vi "AnimateIntersection.vi"() -> ()   [LabVIEW 2022 SP3]
uses:
  <vilib>/Platform/NI_3dgraph.lvlib
panel:
  in  "delay":u32=10
  in  "Type Int":u16(ring) items=["Circle", "Plane"]
  in  "file name":string
  in  "save image":bool
  out "frame#":i32
  in  "Variables":T1={"sound spd (cm/s)"=150000, "time step (s)"=5e-07} {"time step (s)" format="%.2e"}
  in  "rotate P to -y":bool
  in  "Ring":i32(ring)=3 items=["Spherical cap", "Center Strip", "Half Sphere", "Wedge"]
  out "Output Cluster":T2 {"r5" format="%.2f"; "r4" format="%.4f"; "r3" format="%.4f"; "r2" format="%.4f"; "r1" format="%.4f"; "r0" format="%.2f"}
  in  "strip":cluster{"radius":dbl, "h":dbl, "a":dbl}={"radius"=4.0, "h"=0.5, "a"=3.0} {"radius" format="%.2f"; "a" format="%.2f"; "h" format="%.2f"}
  in  "P":cluster{"x":dbl, "y":dbl, "z":dbl}={"x"=0.2, "y"=-1.0, "z"=0.2} {"x" format="%.2f"; "z" format="%.2f"; "y" format="%.2f"}
  in  "ct sphere":cluster{"radius":dbl, "theta":dbl, "phi":dbl}={"radius"=10.0, "theta"=160.0, "phi"=100.0} {"radius" format="%.2f"; "phi" format="%.2f"; "theta" format="%.2f"}
  in  "3D Parametric Surface":refnum<k7>(container)
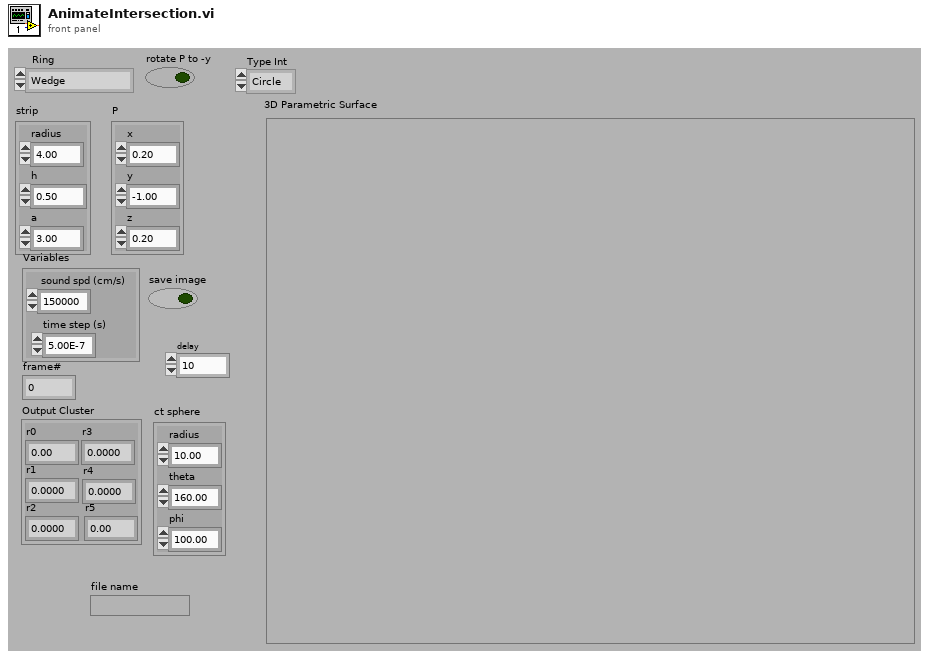
[diagram p1: front panel]
types:
  T1 = cluster{"sound spd (cm/s)":i32, "time step (s)":sgl}
  T2 = cluster{"r0":dbl, "r1":dbl, "r2":dbl, "r3":dbl, "r4":dbl, "r5":dbl}
  T3 = cluster{"r (cm)":dbl, "phih":dbl, "thetaw":dbl, "A":dbl, "B":dbl, "Dtemp":dbl}
  T4 = cluster{"alpha":bool, "beta":bool, "theta":bool, "phi":bool}
  T5 = typedef "LVRectTypeDef.ctl" = cluster{"left":i16, "top":i16, "right":i16, "bottom":i16}
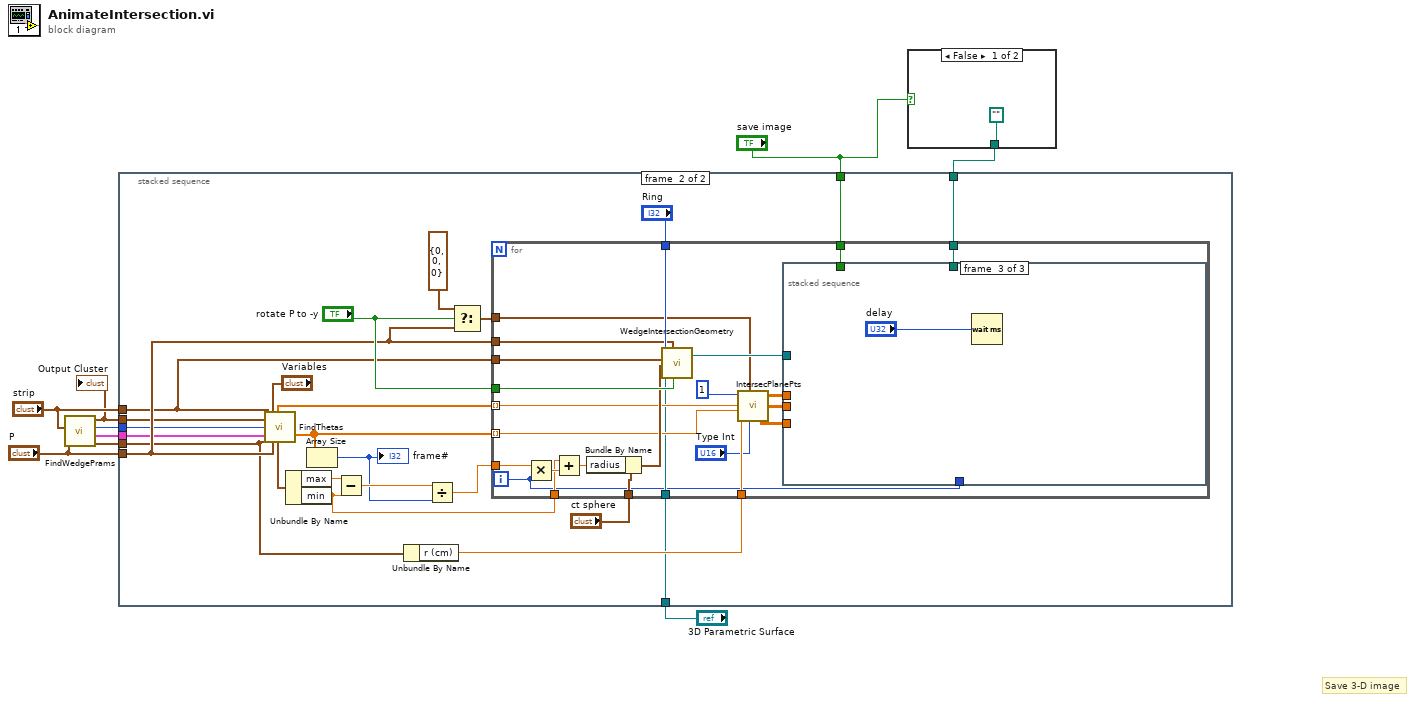
[diagram p0: block diagram]
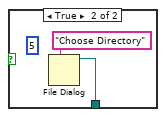
[diagram p2: hidden frame]
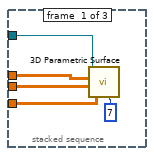
[diagram p4: hidden frame]
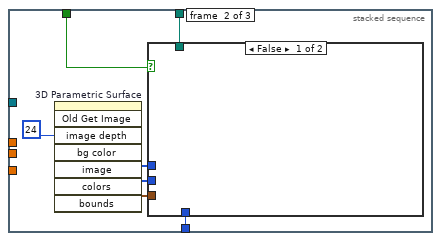
[diagram p5: hidden frame]
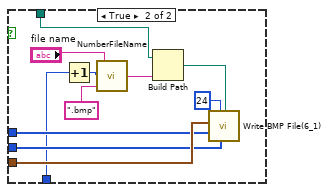
[diagram p6: hidden frame]
diagram:
  # "Save 3-D image"
  n1 = call "FindWedgePrams.vi"("P"="P", "strip"="strip") -> ("variables"=w4:T3, "Location Tests"=w6:T4, "Case Number"=w5:i32, "r values (cm)"=w3:T2)  [unwired: 2 in, 1 out]
  "Output Cluster" <- w3
  n2 = case shown="False" "save image" {
    tunnel: [path "" w11] -> w1
    frame False {
    }
    frame True {
      (unwired) 5
      n3 = File Dialog(7:"Choose Directory") -> (3:w11:path)  [unwired: 6 in, 3 out]
    }
  }
  n4 = stacked-sequence {
    tunnel: "P" -> [_ w22]
    tunnel: "strip" -> [_ w20]
    tunnel: "3D Parametric Surface" -> [_ w19]
    tunnel: w3 -> [_ w18]
    tunnel: w6 -> [_ w17]
    tunnel: w5 -> [_ w16]
    tunnel: w4 -> [_ w15]
    tunnel: "save image" -> [_ w14]
    tunnel: w1 -> [_ w13]
    frame #0 {
    }
    frame #1 {
      n5 = call "FindThetas.vi"("strip"=w20, "r values (cm)"=w18, "Case Number"=w16, "Location Tests"=w17, "P constants"=w15, "Variables"="Variables", "P (cm)"=w22) -> ("d"=w31:dbl[], "min/max r"=w36:cluster{"max":dbl, "min":dbl}, "sigma"=w30:dbl[])  [unwired: 2 in, 8 out]
      n6 = Unbundle By Name(w36) -> ("max"=w35:dbl, "min"=w32:dbl)
      n7 = Array Size(array=w30) -> (size(s)=w27:i32)
      "frame#" <- w27
      n8 = Subtract(x=w35, y=w32) -> (x-y=w34:dbl)
      n9 = Unbundle By Name(w15) -> ("r (cm)"=w21:dbl)
      n10 = Divide(x=w34, y=w27) -> (x/y=w33:dbl)
      n11 = Select(t=cluster{"radius":i32, "theta":i32, "phi":i32} {"radius"=0, "theta"=0, "phi"=0} ("ct sphere"), s="rotate P to -y", f=w22) -> (s? t:f=w29:cluster{"x":dbl, "y":dbl, "z":dbl})
      n12 = for {
        tunnel: w33 -> [w60]
        tunnel: w32 -> [w58]
        tunnel: w31 -> [w47] mode=indexing
        tunnel: w21 -> [w46]
        tunnel: w30 -> [w48] mode=indexing
        tunnel: w29 -> [w49]
        tunnel: "Ring" -> [w57]
        tunnel: w22 -> [w56]
        tunnel: w20 -> [w55]
        tunnel: "rotate P to -y" -> [w54]
        tunnel: "ct sphere" -> [w53]
        tunnel: w19 -> [w41]
        tunnel: w14 -> [w39]
        tunnel: w13 -> [w38]
        i -> [w40]
        n13 = Multiply(x=w60, y=w40) -> (x*y=w59:dbl)
        n14 = Add(x=w58, y=w59) -> (x+y=w52:dbl)
        n15 = Bundle By Name(cluster=w53, "radius"=w52) -> (w51:cluster{"radius":dbl, "theta":dbl, "phi":dbl})
        n16 = call "WedgeIntersectionGeometry.vi"("rotate P to -y"=w54, "P"=w56, "3D Parametric Surface"=w41, "ct sphere"=w51, "strip"=w55, "Ring"=w57) -> ("3D graph out"=w50:refnum<k7>)  [unwired: 1 in]
        n17 = call "IntersecPlanePts.vi"("circles"=1, "P"=w49, "d"=w47, "Sigma"=w48, "Ring"="Type Int", "r"=w46) -> ("x matrix"=w45:dbl[][], "y matrix"=w44:dbl[][], "z matrix"=w43:dbl[][])
        n18 = stacked-sequence {
          tunnel: w50 -> [w64 _ _]
          tunnel: w45 -> [w63 _ _]
          tunnel: w44 -> [w62 _ _]
          tunnel: w43 -> [w61 _ _]
          tunnel: w40 -> [_ w68 _]
          tunnel: w39 -> [_ w67 _]
          tunnel: w38 -> [_ w66 _]
          frame #0 {
            n19 = call <vilib>:"3D Parametric Surface.vi"("plot number (1)"=7, "z matrix"=w61, "y matrix"=w62, "x matrix"=w63, "3D graph"=w64) -> ()  [unwired: 5 in, 2 out]
          }
          frame #1 {
            n20 = invoke on="3D Parametric Surface" class="AXCont" method="Old Get Image"("image depth"=24) -> ("image"=w71:u8[], "colors"=w70:u32[], "bounds"=w69:T5)  [unwired: 7 in, 5 out]
            n21 = case shown="False" w67 {
              tunnel: w69 -> [_ w82]
              tunnel: w70 -> [_ w81]
              tunnel: w71 -> [_ w80]
              tunnel: w68 -> [_ w75]
              tunnel: w66 -> [_ w74]
              frame False {
              }
              frame True {
                n22 = Increment(x=w75) -> (x+1=w77:i32)
                n23 = call "NumberFileName.vi"("String"=".bmp", "File number"=w77, "file name"="file name") -> ("Numbered File"=w78:string)
                n24 = Build Path(base path=w74, name or relative path=w78) -> (appended path=w73:path)
                n25 = call <vilib>:"Write BMP File(6_1).vi"("color table"=w81, "depth"=24, "flattened image data"=w80, "rect"=w82, "path to BMP file"=w73) -> ()  [unwired: 5 in, 2 out]
              }
            }
          }
          frame #2 {
            n26 = Wait (ms)(milliseconds to wait="delay") -> ()  [unwired: 1 out]
          }
        }
      }
    }
  }
